vi "Validate Arguments.vi"(8 "error in (no error)":errorcluster, 11 "CLIAction in":refnum<class "CLIAction.lvclass">) -> (0 "error out":errorcluster, 2 "Problems":string[](array[string]), 3 "CLIAction out":refnum<class "CLIAction.lvclass">)   [LabVIEW 2020, in "GPackTools.lvlib" / "CLIAction.lvclass"]
uses:
  CLIAction.lvclass
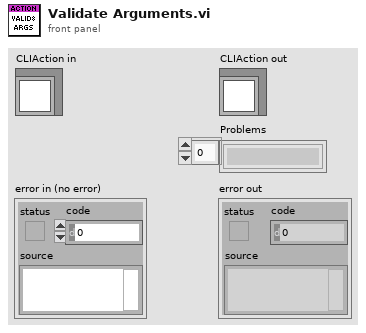
[diagram p1: front panel]
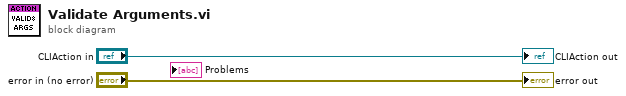
[diagram p0: block diagram]
diagram:
  "error out" <- "error in (no error)"
  "CLIAction out" <- "CLIAction in"
